vi "Create Zip File.vi"() -> ()   [LabVIEW 2023]
doc: "This VI will zip up a source directory into a Zip file."
panel:
  out "Generated Zip File":path
  # "Overview: Demonstrates the use of the Zip VIs to generate a Zip file.\nInstructions:\n1. Run this VI. It will create a Zip file containing the contents of [LabVIEW]\\examples\\Synchronization.\n2. Open the Zip file displayed in the Generated Zip File path below. It should contain the contents of the Synchronization examples folder.\n3. Delete the Zip file (located at [LabVIEW Data]\\Example Zip File.zip) when you are done."
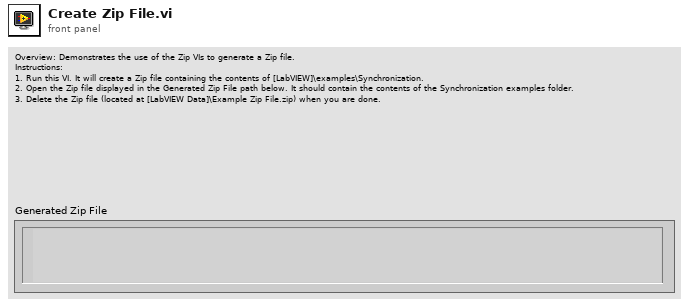
[diagram p1: front panel]
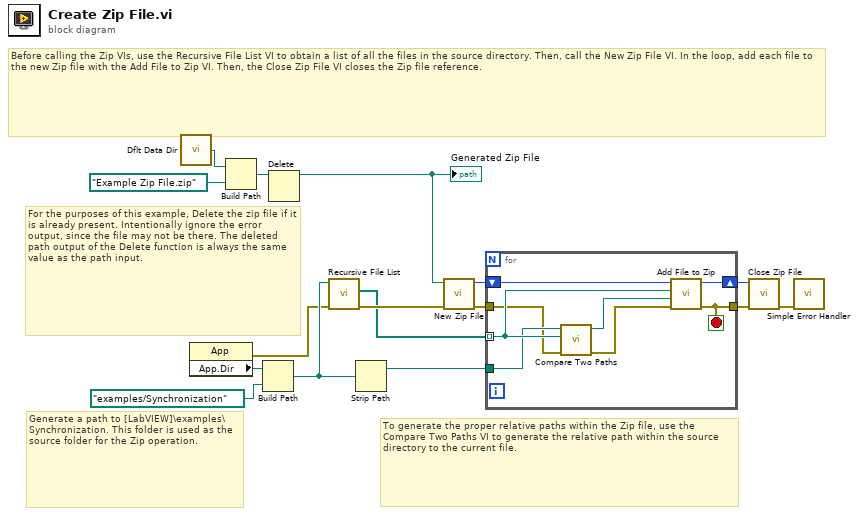
[diagram p0: block diagram]
diagram:
  # "Generate a path to [LabVIEW]\\examples\\Synchronization. This folder is used as the source folder for the Zip operation."
  # "To generate the proper relative paths within the Zip file, use the Compare Two Paths VI to generate the relative path within the source directory to the current file."
  # "For the purposes of this example, Delete the zip file if it is already present. Intentionally ignore the error output, since the file may not be there. The deleted path output of the Delete function is always the same value as the path input."
  # "Before calling the Zip VIs, use the Recursive File List VI to obtain a list of all the files in the source directory. Then, call the New Zip File VI. In the loop, add each file to the new Zip file with the Add File to Zip VI. Then, the Close Zip File VI closes the Zip file reference."
  n1 = call <vilib>:"Dflt Data Dir.vi"() -> ("App:Default Data Directory"=w5:path)
  n2 = property class="App"() -> (error out=w2:errorcluster, "App.Dir"=w9:path)  [unwired: 2 in, 1 out]
  n3 = Build Path(base path=w5, name or relative path=path "Example Zip File.zip" ("default name")) -> (appended path=w4:path)
  n4 = Build Path(base path=w9, name or relative path=path "examples/Synchronization") -> (appended path=w8:path)
  n5 = Delete(path (use dialog)=w4) -> (deleted path=w3:path)  [unwired: 4 in, 2 out]
  "Generated Zip File" <- w3
  n6 = call <vilib>:"Recursive File List.vi"("error in (no error)"=w2, "Folder Path"=w8) -> ("error out"=w11:errorcluster, "All Files in Dir"=w10:path[])  [unwired: 5 in, 3 out]
  n7 = Strip Path(path=w8) -> (stripped path=w1:path)  [unwired: 1 out]
  n8 = call <vilib>:"New Zip File.vi"("error in (no error)"=w11, "target"=w3) -> ("error out"=w14:errorcluster, "zip file out"=w15:i64)  [unwired: 1 in, 3 out]
  n9 = for {
    tunnel: w10 -> [w21] mode=indexing
    tunnel: w14 -> [w18]
    tunnel: [w22] -> w13
    shift-right: [w23] -> w12
    shift-left: w15 -> [w24]
    tunnel: w1 -> [w20]
    stop <- w22 stop-if-true
    n10 = call <vilib>:"Compare Two Paths.vi"("error in (no error)"=w18, "Path 2"=w21, "Path 1"=w20) -> ("error out"=w17:errorcluster, "Relative Path from 1 to 2"=w19:path)  [unwired: 5 in, 2 out]
    n11 = call <vilib>:"Add File to Zip.vi"("error in (no error)"=w17, "destination path in zip"=w19, "source file path"=w21, "zip file in"=w24) -> ("error out"=w22:errorcluster, "zip file out"=w23:i64)  [unwired: 6 out]
  }
  n12 = call <vilib>:"Close Zip File.vi"("error in (no error)"=w13, "zip file in"=w12) -> ("error out"=w16:errorcluster)  [unwired: 1 in, 4 out]
  n13 = call <vilib>:"Simple Error Handler.vi"("error in (no error)"=w16) -> ()  [unwired: 1 in, 8 out]
